vi "ServoSub!.vi"(6 "freq [Hz] 2":dbl=50.0, 9 "position [%FS] 2":dbl(slide) scale=-200.0..200.0, 10 "freq [Hz]":dbl=50.0, 11 "position [%FS]":dbl(slide) scale=-200.0..200.0) -> (1 "Numeric":dbl, 2 "freq [Hz] 4":dbl, 3 "Numeric 2":dbl, 4 "freq [Hz] 3":dbl)   [LabVIEW 2018]
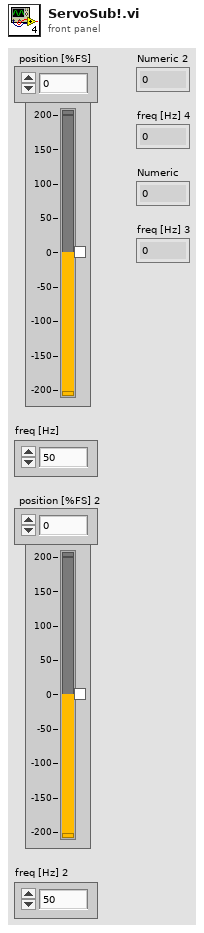
[diagram p1: front panel]
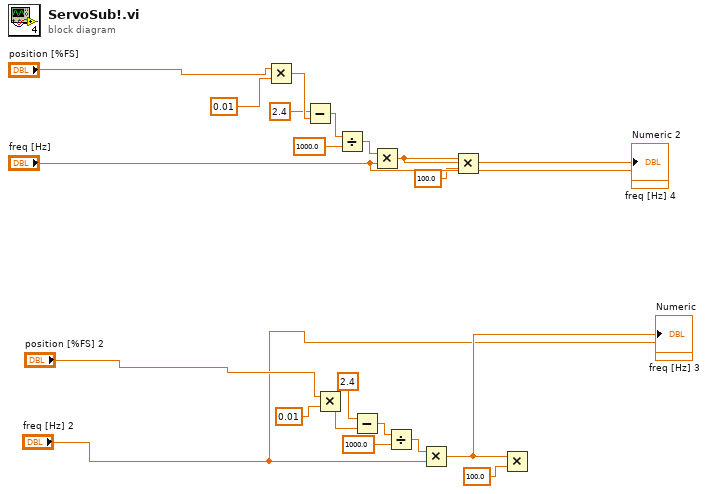
[diagram p0: block diagram]
diagram:
  n1 = Multiply(x="position [%FS]", y=0.01) -> (x*y=w18:dbl)
  n2 = Subtract(x=2.4 ("y"), y=w18) -> (x-y=w2:dbl)
  n3 = Multiply(x="position [%FS] 2", y=0.01) -> (x*y=w20:dbl)
  n4 = Divide(x=w2, y=1000.0) -> (x/y=w4:dbl)
  n5 = Subtract(x=2.4 ("y"), y=w20) -> (x-y=w12:dbl)
  n6 = Multiply(x=w4, y="freq [Hz]") -> (x*y=w7:dbl)
  "Numeric 2" <- w7
  n7 = Divide(x=w12, y=1000.0) -> (x/y=w10:dbl)
  n8 = Multiply(x=w10, y="freq [Hz] 2") -> (x*y=w14:dbl)
  "Numeric" <- w14
  n9 = Multiply(x=w7, y=100.0) -> ()  [unwired: 1 out]
  n10 = Multiply(x=w14, y=100.0) -> ()  [unwired: 1 out]
  "freq [Hz] 3" <- "freq [Hz] 2"
  "freq [Hz] 4" <- "freq [Hz]"
